vi "File_INI Read Write Name Value Array.vi"(6 "Read(f) Write(t)":bool, 7 "Section Name":string, 8 "Error":errorcluster, 9 "File Path":path, 11 "Name Data Array":string[][](array[string])) -> (0 "Error Out":errorcluster, 3 "Name Data Array Out":string[][](array[string]))   [LabVIEW 2020]
uses:
  <vilib>/Utility/config.llb/Write Key (String).vi
  <vilib>/Utility/config.llb/Read Key (String).vi
  <vilib>/Utility/file.llb/Read Delimited Spreadsheet (string).vi
  <vilib>/Utility/file.llb/Write Delimited Spreadsheet (string).vi
  <vilib>/Utility/config.llb/NI_LVConfig.lvlib
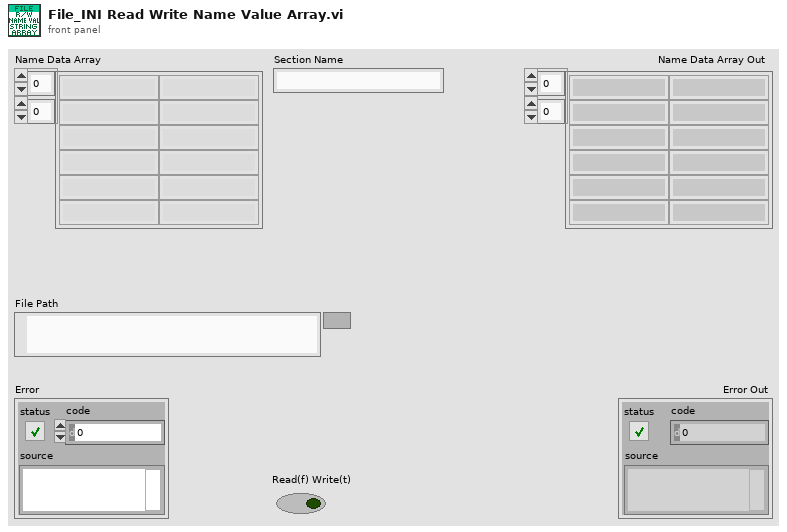
[diagram p1: front panel]
types:
  T1 = typedef "NI_LVConfig.lvlib/Config Data RefNum.ctl" = refnum<k1>
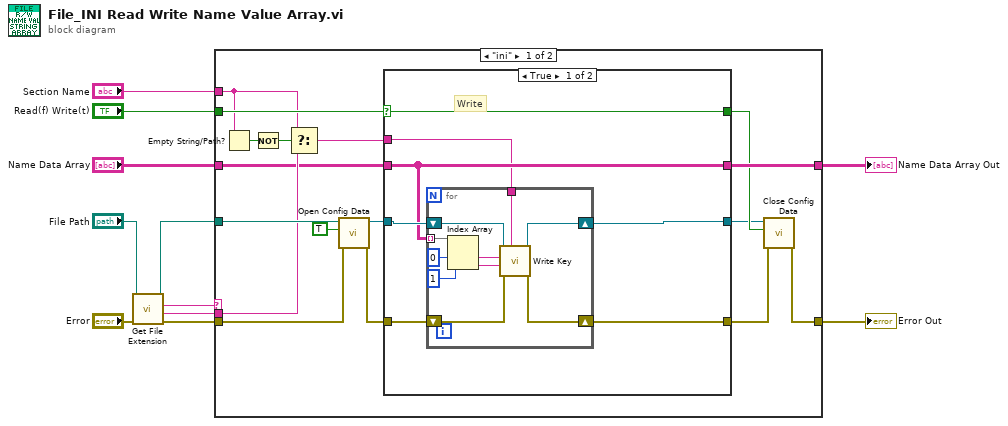
[diagram p0: block diagram]
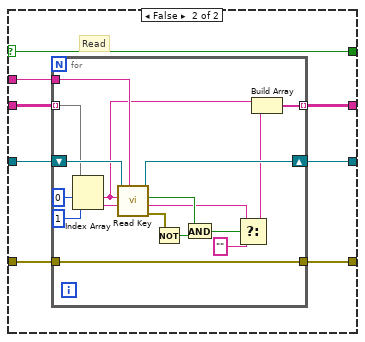
[diagram p2: hidden frame]
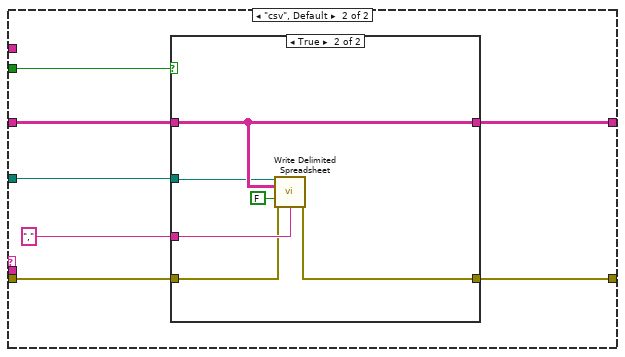
[diagram p3: hidden frame]
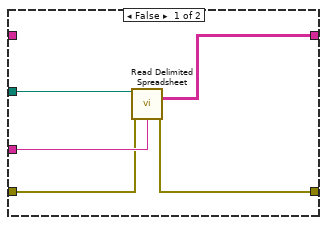
[diagram p4: hidden frame]
diagram:
  n1 = call <vilib>:"Get File Extension.vi"("error in (no error)"="Error", "file"="File Path") -> ("error out"=w4:errorcluster, "filename without extension"=w3:string, "lowercase file extension"=w6:string, "dup file"=w5:path)  [unwired: 5 in, 1 out]
  n2 = case shown="\"ini\"" w6 {
    tunnel: "Name Data Array" -> [w15 w77]
    tunnel: [w14 w76] -> w10
    tunnel: [w25 w75] -> w9
    tunnel: "Read(f) Write(t)" -> [w24 w74]
    tunnel: w4 -> [w26 w73]
    tunnel: w5 -> [w28 w72]
    tunnel: "Section Name" -> [w21 _]
    tunnel: w3 -> [w19 _]
    frame "ini" {
      n3 = Empty String/Path?(string/path=w21) -> (empty?=w23:bool)
      n4 = Not(x=w23) -> (.not. x?=w22:bool)
      n5 = Select(t=w21, s=w22, f=w19) -> (s? t:f=w20:string)
      n6 = call <vilib>:"Open Config Data.vi"("error in (no error)"=w26, "create file if necessary (T)"=TRUE, "configuration file path"=w28) -> ("error out"=w18:errorcluster, "refnum"=w16:T1)  [unwired: 6 in, 1 out]
      n7 = case shown="True" w24 {
        selector: w24 -> [w35 w53]
        tunnel: w20 -> [w29 w48]
        tunnel: w18 -> [w32 w50]
        tunnel: [w31 w49] -> w17
        tunnel: w16 -> [w34 w52]
        tunnel: w15 -> [w30 w47]
        tunnel: [w30 w46] -> w14
        tunnel: [w35 w53] -> w13
        tunnel: [w33 w51] -> w12
        frame True {
          # "Write"
          n8 = for {
            shift-right: [w44] -> w33
            shift-left: w34 -> [w45]
            shift-right: [w42] -> w31
            shift-left: w32 -> [w43]
            tunnel: w30 -> [w41] mode=indexing
            tunnel: w29 -> [w36]
            n9 = Index Array(array=w41, index #1=0 ("index"), index #2=1 ("index")) -> (element #1=w38:string, element #2=w37:string)
            n10 = call-poly <vilib>:"Write Key.vi"("section"=w36, "error in (no error)"=w43, "value"=w37, "key"=w38, "refnum"=w45) -> ("error out"=w42:errorcluster, "refnum out"=w44:T1)  [unwired: 4 in, 1 out]
          }
        }
        frame False {
          # "Read"
          n11 = for {
            shift-right: [w69] -> w51
            shift-left: w52 -> [w70]
            tunnel: w47 -> [w68] mode=indexing
            tunnel: w48 -> [w65]
            tunnel: [w62] -> w46 mode=indexing
            tunnel: w50 -> [w61]
            tunnel: [w61] -> w49
            n12 = Index Array(array=w68, index #1=0 ("index"), index #2=1 ("index")) -> (element #1=w63:string, element #2=w64:string)
            n13 = call-poly <vilib>:"Read Key.vi"("section"=w65, "default value"=w64, "key"=w63, "refnum"=w70) -> ("error out"=w60:errorcluster, "value"=w55:string, "found?"=w57:bool, "refnum out"=w69:T1)  [unwired: 4 in]
            n14 = Not(x=w60) -> (.not. x?=w58:bool)
            n15 = And(x=w57, y=w58) -> (x .and. y?=w59:bool)
            n16 = Select(t=w55, s=w59, f="") -> (s? t:f=w54:string)
            n17 = Build Array(w63, w54) -> (w62:string[])
          }
        }
      }
      n18 = call <vilib>:"Close Config Data.vi"("error in (no error)"=w17, "write file if changed (T)"=w13, "refnum"=w12) -> ("error out"=w25:errorcluster)  [unwired: 7 in, 1 out]
    }
    frame "csv", Default {
      n19 = case shown="True" w74 {
        tunnel: w77 -> [_ w88]
        tunnel: [w81 w88] -> w76
        tunnel: w73 -> [w79 w84]
        tunnel: [w78 w83] -> w75
        tunnel: w72 -> [w82 w86]
        tunnel: "," ("delimiter (\\t)") -> [w80 w87]
        frame False {
          n20 = call-poly <vilib>:"Read Delimited Spreadsheet.vi"("file path (dialog if empty)"=w82, "error in (no error)"=w79, "delimiter (\\t)"=w80) -> ("all rows"=w81:string[][], "error out"=w78:errorcluster)  [unwired: 7 in, 4 out]
        }
        frame True {
          n21 = call-poly <vilib>:"Write Delimited Spreadsheet.vi"("file path (dialog if empty)"=w86, "2D data"=w88, "append to file? (new file:F)"=FALSE ("append to file? (F)"), "error in (no error)"=w84, "delimiter (\\t)"=w87) -> ("error out"=w83:errorcluster)  [unwired: 9 in, 1 out]
        }
      }
    }
  }
  "Name Data Array Out" <- w10
  "Error Out" <- w9
